vi "User - Get Info.vi"(6 "Info State":T1=enum."Access Level", 8 "Error In":errorcluster, 11 "Username:":string) -> (0 "Error Out":errorcluster, 3 "Data Out":string)   [LabVIEW 2020]
uses:
  Control/Header - User Management.ctl
  Control/State - FGV.ctl
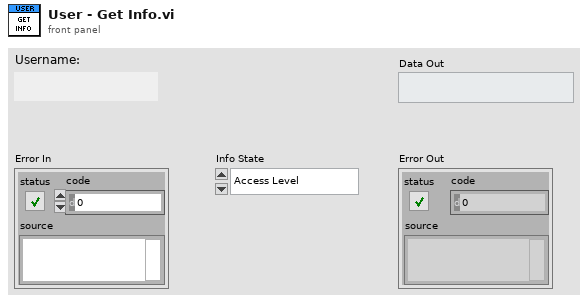
[diagram p1: front panel]
types:
  T1 = typedef "Header - User Management.ctl" = enum16{"Name", "Staff ID", "Username", "Password", "Access Level", "Status", "Access Page"}
  T2 = typedef "State - FGV.ctl" = enum16{"Write", "Read"}
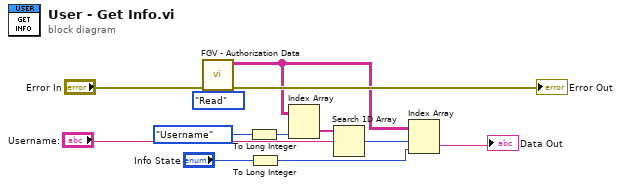
[diagram p0: block diagram]
diagram:
  n1 = call "FGV - Authorization Data.vi"("State - FGV"=State_-_FGV."Read", "Error In"="Error In") -> ("Error Out"=→"Error Out":errorcluster, "Data Out"=w8:string[][])  [unwired: 8 in]
  n2 = To Long Integer(number=Header_-_User_Management."Username" ("Header - User Management")) -> (32bit integer=w6:i32)
  n3 = To Long Integer(number="Info State") -> (32bit integer=w3:i32)
  n4 = Index Array(array=w8, index (col)=w6) -> (element=w9:string[])  [unwired: 1 in]
  n5 = Search 1D Array(1D array=w9, element="Username:") -> (index of element=w5:i32)  [unwired: 1 in]
  n6 = Index Array(array=w8, index (row)=w5, index (col)=w3) -> (element=→"Data Out":string)
